vi "Read Error Status.vi"(8 "error in (no error)":errorcluster, 11 "MKS MF1 in":refnum<class "PL MKS MF1 USB.lvclass">) -> (0 "error out":errorcluster, 2 "error status":T1, 3 "MKS MF1 out":refnum<class "PL MKS MF1 USB.lvclass">)   [LabVIEW 2015, in "PL MKS MF1 USB.lvclass"]
doc: "Reads device error status."
uses:
  PL MKS MF1 USB.lvclass
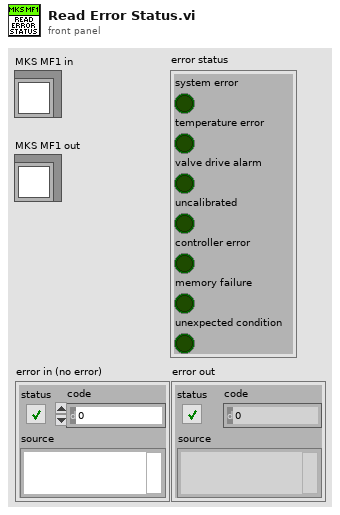
[diagram p1: front panel]
types:
  T1 = cluster{"system error":bool, "temperature error":bool, "valve drive alarm":bool, "uncalibrated":bool, "controller error":bool, "memory failure":bool, "unexpected condition":bool}
  T2 = cluster{"[0]":bool, "[1]":bool, "[2]":bool, "[3]":bool, "[4]":bool, "[5]":bool, "[6]":bool}
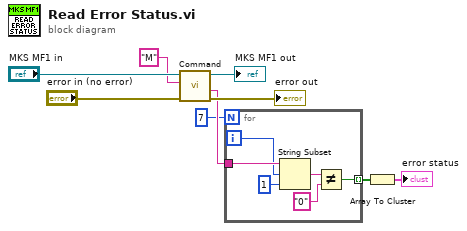
[diagram p0: block diagram]
diagram:
  n1 = call "Command.vi"("error in (no error)"="error in (no error)", "command"="M", "MKS MF1 in"="MKS MF1 in") -> ("error out"=→"error out":errorcluster, "response value"=w4:string, "MKS MF1 out"=→"MKS MF1 out":refnum<class "PL MKS MF1 USB.lvclass">)  [unwired: 5 in, 1 out]
  n2 = for {
    N: 7 -> [_]
    tunnel: w4 -> [w15]
    tunnel: [w10] -> w3 mode=indexing
    i -> [w11]
    n3 = String Subset(string=w15, offset (0)=w11, length (rest)=1 ("length (rest)")) -> (substring=w13:string)
    n4 = Not Equal?(x=w13, y="0") -> (x != y?=w10:bool)
  }
  n5 = Array To Cluster(array=w3) -> (cluster=→"error status":T2)
